vi "Swerve Dance Teleop Emulator.vi"(8 "dt":dbl, 9 "Current Heading":dbl, 10 "Operator ID":refnum<k1>, 11 "Driver ID":refnum<k1>) -> (3 "Robot Velocities":T3)   [LabVIEW 2020]
uses:
  <vilib>/Analysis/NI_AALPro.lvlib
  <vilib>/Analysis/coordinate.llb/2D Cartesian Coordinate Rotation (Array).vi
  swerve/Type Definitions/Data/Robot Velocities.ctl
panel:
  in  "Controls Type":T1(ring)
  in  "Velo Limits":T2
  in  "Max Deltas":cluster{"dx":dbl, "dy":dbl, "dtheta":dbl}={"dx"=10.0, "dy"=10.0, "dtheta"=180.0}
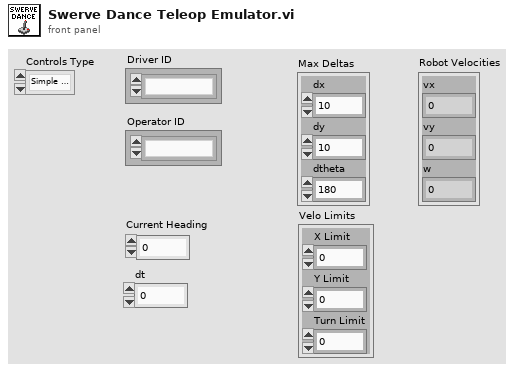
[diagram p1: front panel]
types:
  T1 = enum16{"Simple Offset Control", "Velocity Limited v1", "Center of Rotation v1"}
  T2 = cluster{"X Limit":dbl, "Y Limit":dbl, "Turn Limit":dbl}
  T3 = typedef "Robot Velocities.ctl" = cluster{"vx":dbl, "vy":dbl, "w":dbl}
  T4 = cluster{"X axis":i32, "Y axis":i32, "Z axis":i32, "X axis rotation":i32, "Y axis rotation":i32, "Z axis rotation":i32, "U axis":i32, "V axis":i32}
  T5 = cluster{"X axis":dbl, "Y axis":dbl, "Z axis":dbl, "X axis rotation":dbl, "Y axis rotation":dbl, "Z axis rotation":dbl, "U axis":dbl, "V axis":dbl}
  T6 = cluster{"X axis":dbl, dbl, "X axis rotation":dbl}
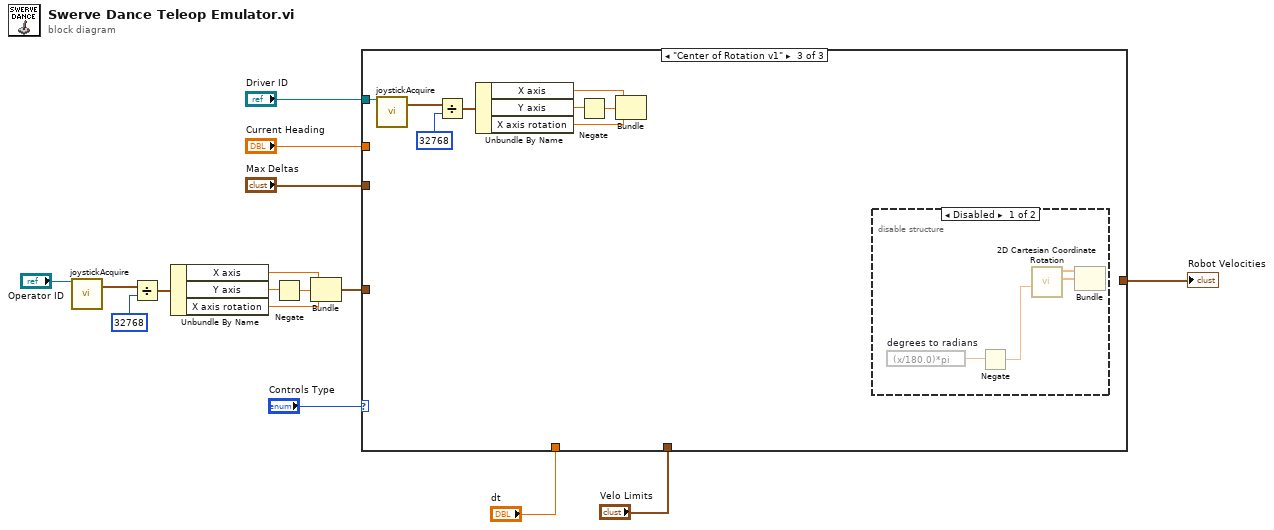
[diagram p0: block diagram]
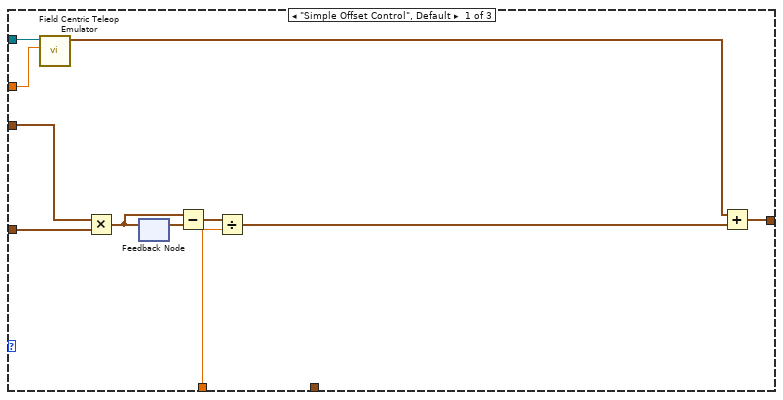
[diagram p2: hidden frame]
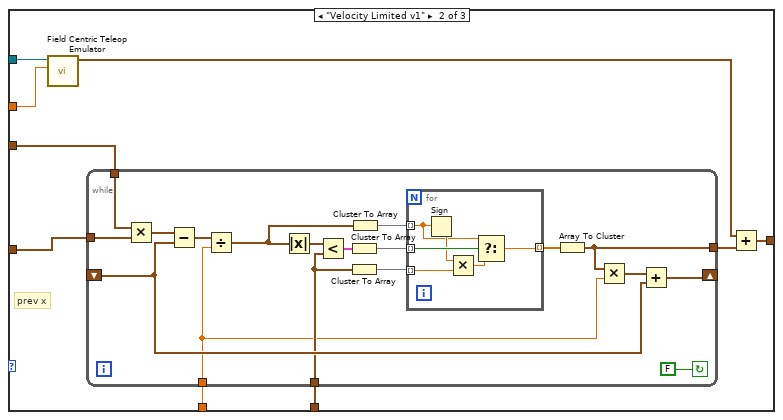
[diagram p3: hidden frame]
diagram:
  n1 = call <vilib>:"joystickAcquire.vi"("device ID"="Operator ID") -> ("axis info"=w16:T4)  [unwired: 14 in, 4 out]
  n2 = Divide(x=w16, y=32768 ("X axis")) -> (x/y=w14:T5)
  n3 = Unbundle By Name(w14) -> ("X axis"=w12:dbl, "Y axis"=w10:dbl, "X axis rotation"=w11:dbl)
  n4 = Negate(x=w10) -> (-x=w9:dbl)
  n5 = Bundle("X axis"=w12, w9, "X axis rotation"=w11) -> (w6:T6)  [unwired: 1 in]
  n6 = case shown="\"Center of Rotation v1\"" "Controls Type" {
    tunnel: "Max Deltas" -> [w24 w36 _]
    tunnel: "dt" -> [w23 w35 _]
    tunnel: w6 -> [w17 w34 _]
    tunnel: "Velo Limits" -> [_ w33 _]
    tunnel: [w20 w28 _] -> w1
    tunnel: "Current Heading" -> [w22 w32 _]
    tunnel: "Driver ID" -> [w21 w31 w61]
    frame "Simple Offset Control", Default {
      n7 = call "Field Centric Teleop Emulator.vi"("Current Heading"=w22, "device ID"=w21) -> ("Robot Velocities"=w19:T3)  [unwired: 9 in]
      n8 = Multiply(x=w24, y=w17) -> (x*y=w26:cluster{dbl, dbl, dbl})
      n9 = feedback #1() -> (w27:cluster{dbl, dbl, dbl})  [unwired: 1 in]
      n10 = feedback-in #1(w26) -> ()
      n11 = Subtract(x=w26, y=w27) -> (x-y=w25:cluster{dbl, dbl, dbl})
      n12 = Divide(x=w25, y=w23) -> (x/y=w18:cluster{dbl, dbl, dbl})
      n13 = Add(x=w19, y=w18) -> (x+y=w20:T3)
    }
    frame "Velocity Limited v1" {
      # "prev x"
      n14 = call "Field Centric Teleop Emulator.vi"("Current Heading"=w32, "device ID"=w31) -> ("Robot Velocities"=w29:T3)  [unwired: 9 in]
      n15 = while {
        shift-right: [w43] -> _
        shift-left: _ -> [w44]
        tunnel: w34 -> [w47]
        tunnel: w33 -> [w40]
        tunnel: w36 -> [w46]
        tunnel: w35 -> [w38]
        tunnel: [w39] -> w30
        stop <- FALSE continue-if-true
        n16 = Multiply(x=w46, y=w47) -> (x*y=w45:cluster{dbl, dbl, dbl})
        n17 = Subtract(x=w45, y=w44) -> (x-y=w42:cluster{dbl, dbl, dbl})
        n18 = Divide(x=w42, y=w38) -> (x/y=w41:cluster{dbl, dbl, dbl})
        n19 = Absolute Value(x=w41) -> (abs(x)=w49:cluster{dbl, dbl, dbl})
        n20 = Less?(x=w49, y=w40) -> (x < y?=w54:cluster{bool, bool, bool})
        n21 = Cluster To Array(cluster=w54) -> (array=w53:bool[])
        n22 = Cluster To Array(cluster=w40) -> (array=w51:dbl[])
        n23 = Cluster To Array(cluster=w41) -> (array=w52:dbl[])
        n24 = for {
          tunnel: w53 -> [w60] mode=indexing
          tunnel: w52 -> [w57] mode=indexing
          tunnel: w51 -> [w59] mode=indexing
          tunnel: [w55] -> w50 mode=indexing
          n25 = Sign(1:w57) -> (0:w58:dbl)
          n26 = Multiply(x=w58, y=w59) -> (x*y=w56:dbl)
          n27 = Select(t=w57, s=w60, f=w56) -> (s? t:f=w55:dbl)
        }
        n28 = Array To Cluster(array=w50) -> (cluster=w39:cluster{"[0]":dbl, "[1]":dbl, "[2]":dbl})
        n29 = Multiply(x=w39, y=w38) -> (x*y=w37:cluster{"[0]":dbl, "[1]":dbl, "[2]":dbl})
        n30 = Add(x=w37, y=w44) -> (x+y=w43:cluster{"[0]":dbl, "[1]":dbl, "[2]":dbl})
      }
      n31 = Add(x=w29, y=w30) -> (x+y=w28:T3)
    }
    frame "Center of Rotation v1" {
      n32 = call <vilib>:"joystickAcquire.vi"("device ID"=w61) -> ("axis info"=w68:T4)  [unwired: 14 in, 4 out]
      n33 = Divide(x=w68, y=32768 ("X axis")) -> (x/y=w66:T5)
      n34 = Unbundle By Name(w66) -> ("X axis"=w65:dbl, "Y axis"=w63:dbl, "X axis rotation"=w64:dbl)
      n35 = Negate(x=w63) -> (-x=w62:dbl)
      n36 = Bundle("X axis"=w65, w62, "X axis rotation"=w64) -> ()  [unwired: 1 in, 1 out]
      n37 = disable-structure shown="Disabled" {
        frame Disabled {
          n38 = expression code="(x/180.0)*pi" "degrees to radians"() -> (w72:dbl)  [unwired: 1 in]
          n39 = Negate(x=w72) -> (-x=w71:dbl)
          n40 = call-poly <vilib>:"2D Cartesian Coordinate Rotation.vi"("theta"=w71) -> ("Y Out"=w69:dbl[], "X Out"=w70:dbl[])  [unwired: 8 in, 1 out]
          n41 = Bundle("X Out"=w70, "Y Out"=w69) -> ()  [unwired: 2 in, 1 out]
        }
        frame Enabled {
        }
      }
    }
  }
  "Robot Velocities" <- w1
